vi "Check Terminate on Fail.vi"(8 "error in (no error)":errorcluster, 11 "Tester in":refnum<class "Tester.lvclass">) -> (0 "error out":errorcluster, 2 "Terminate":bool, 3 "Tester out":refnum<class "Tester.lvclass">)   [LabVIEW 2020, in "Tester.lvlib" / "Tester.lvclass"]
uses:
  Tester.lvclass
  Results/Result.ctl
  Tester.lvclass/Tester.ctl
  Results/Results.lvclass
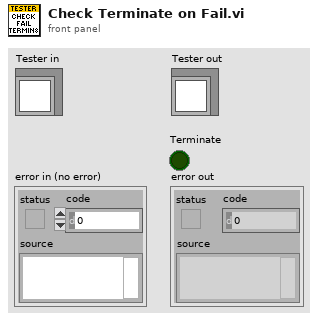
[diagram p1: front panel]
types:
  T1 = typedef "Tester.lvlib/Results.lvclass/Result.ctl" = enum16{"No Result", "Pass", "Fail", "Error", "Abort"}
  T2 = typedef "Tester.lvlib/Tester.lvclass/Config Ref.ctl" = cluster{"Stop on Fail":bool, "Stop on Error":bool}
  T3 = typedef "Tester.lvlib/Tester.lvclass/Execution Ref.ctl" = cluster{"Sequence":refnum<class "Sequence.lvclass">, "Step":i32, "Results":refnum<class "Results.lvclass">, "State":T4, "Run Step VI":refnum<vi>, "Abort":bool}
  T4 = typedef "Tester.lvlib/Tester.lvclass/State.ctl" = enum16{"Idle", "In Progress", "Completed"}
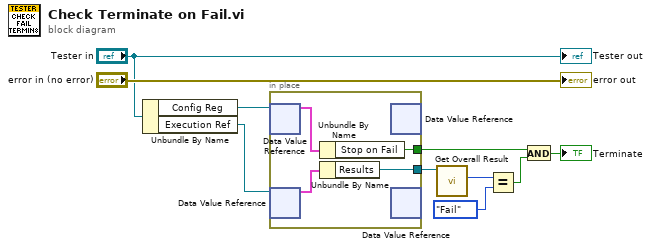
[diagram p0: block diagram]
diagram:
  n1 = Unbundle By Name("Tester in") -> ("Config Reg"=w10:refnum<data-value>, "Execution Ref"=w9:refnum<data-value>)
  n2 = in-place {
    in-place-border: [w13] -> w5
    in-place-border: [w11] -> w8
    n3 = in-place-dvr #1(w10) -> (w14:T2)  [unwired: 1 out]
    n4 = in-place-dvr #2(w9) -> (w12:T3)  [unwired: 1 out]
    n5 = Unbundle By Name(w14) -> ("Stop on Fail"=w13:bool)
    n6 = Unbundle By Name(w12) -> ("Results"=w11:refnum<class "Results.lvclass">)
    n7 = in-place-dvr #1() -> ()  [unwired: 1 in, 2 out]
    n8 = in-place-dvr #2() -> ()  [unwired: 1 in, 2 out]
  }
  n9 = call "Get Overall Result.vi"("Results in"=w8) -> ("Overall Result"=w7:T1)  [unwired: 8 in, 2 out]
  n10 = Equal?(x=w7, y=Result."Fail") -> (x = y?=w4:bool)
  n11 = And(x=w5, y=w4) -> (x .and. y?=→"Terminate":bool)
  "error out" <- "error in (no error)"
  "Tester out" <- "Tester in"
